vi "Find property nodes of cluster.vi"(2 "error in":errorcluster, 3 "Clust Refnum":refnum<vi>) -> (0 "Property Nodes":refnum<vi>[](array[refnum]), 1 "Array of refs to embedded clusters":refnum<vi>[](array[refnum]))   [LabVIEW 2010]
panel:
  out "error out":errorcluster
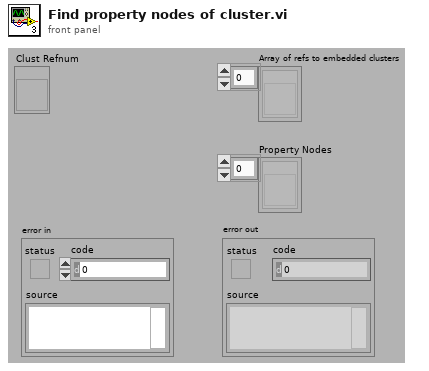
[diagram p1: front panel]
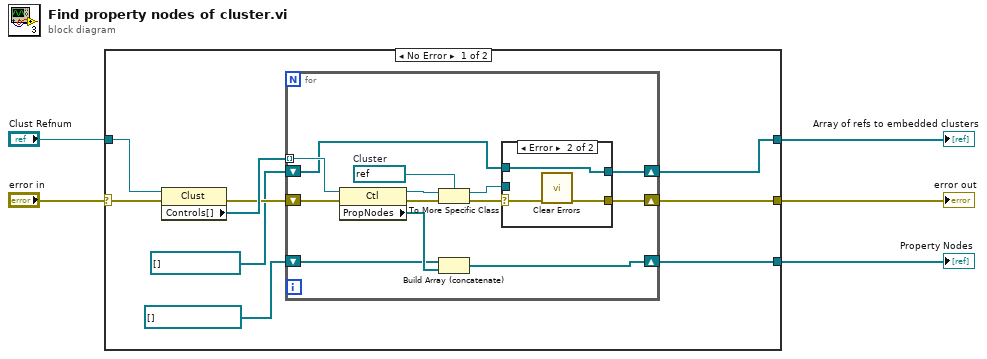
[diagram p0: block diagram]
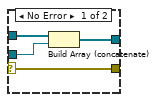
[diagram p2: hidden frame]
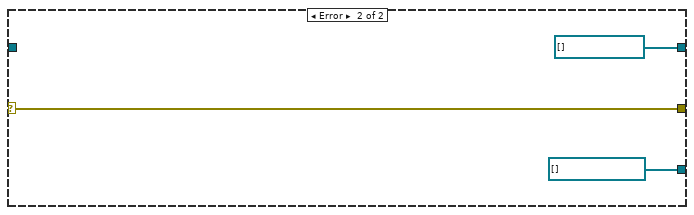
[diagram p3: hidden frame]
diagram:
  n1 = case shown="No Error" "error in" {
    selector: "error in" -> [w12 w35]
    tunnel: "Clust Refnum" -> [w13 _]
    tunnel: [w9 refnum<vi>[] []] -> w4
    tunnel: [w8 refnum<vi>[] []] -> w5
    tunnel: [w6 w35] -> w1
    frame No Error {
      n2 = property class="Clust"(reference=w13, error in=w12) -> (error out=w11:errorcluster, "Controls[]"=w14:refnum<vi>[])  [unwired: 1 out]
      n3 = for {
        tunnel: w14 -> [w27] mode=indexing
        shift-right: [w25] -> w9
        shift-left: refnum<vi>[] [] -> [w23]
        shift-right: [w19] -> w8
        shift-left: refnum<vi>[] [] -> [w20]
        shift-right: [w15] -> w6
        shift-left: w11 -> [w26]
        w22 = refnum<vi> refnum  # Cluster
        n4 = property on="Property Node" class="Ctl"(reference=w27, error in=w26) -> (reference out=w21:refnum<vi>, error out=w16:errorcluster, "PropNodes"=w24:refnum<vi>[])
        n5 = To More Specific Class(target class=w22, reference=w21, error in=w16) -> (specific class reference=w18:refnum<vi>, error out=w17:errorcluster)
        n6 = Build Array (concatenate)(w23, w24) -> (w25:refnum<vi>[])
        n7 = case shown="Error" w17 {
          selector: w17 -> [w28 w33]
          tunnel: w20 -> [w31 w34]
          tunnel: [w30 w34] -> w19
          tunnel: w18 -> [w29 _]
          tunnel: [w28 w32] -> w15
          frame No Error {
            n8 = Build Array (concatenate)(w31, w29) -> (w30:refnum<vi>[])
          }
          frame Error {
            n9 = call <vilib>:"Clear Errors.vi"("error in (no error)"=w33) -> ("error out"=w32:errorcluster)  [unwired: 6 in]
          }
        }
      }
    }
    frame Error {
    }
  }
  "Property Nodes" <- w4
  "Array of refs to embedded clusters" <- w5
  "error out" <- w1
